vi "习题7.2.vi"() -> ()   [LabVIEW 2017]
panel:
  out "波形图":cluster{dbl[]}[](graph)
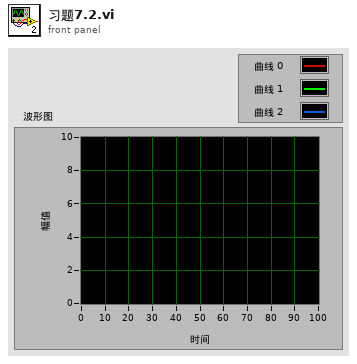
[diagram p1: front panel]
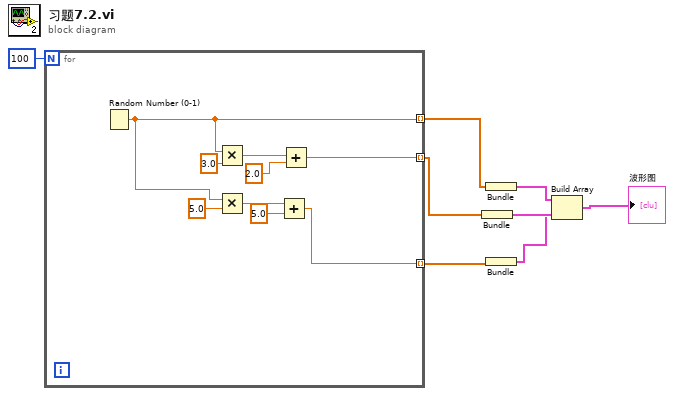
[diagram p0: block diagram]
diagram:
  n1 = for {
    N: 100 -> [_]
    tunnel: [w12] -> w5 mode=indexing
    tunnel: [w11] -> w1 mode=indexing
    tunnel: [w10] -> w4 mode=indexing
    n2 = Random Number (0-1)() -> (number: 0 to 1=w10:dbl)
    n3 = Multiply(x=w10, y=3.0) -> (x*y=w17:dbl)
    n4 = Multiply(x=w10, y=5.0) -> (x*y=w16:dbl)
    n5 = Add(x=w16, y=5.0) -> (x+y=w12:dbl)
    n6 = Add(x=w17, y=2.0) -> (x+y=w11:dbl)
  }
  n7 = Bundle(w1) -> (w7:cluster{dbl[]})  [unwired: 1 in]
  n8 = Bundle(w4) -> (w8:cluster{dbl[]})  [unwired: 1 in]
  n9 = Bundle(w5) -> (w6:cluster{dbl[]})  [unwired: 1 in]
  n10 = Build Array(w8, w7, w6) -> (→"波形图":cluster{dbl[]}[])
